vi "Destructor.vi"(8 "error in":errorcluster, 11 "StringMeasureLimit":refnum<class "StringMeasureLimit.lvclass">) -> (0 "error out":errorcluster)   [LabVIEW 2021, in "ProligentXMLGenerator.lvlib" / "StringMeasureLimit.lvclass"]
uses:
  StringMeasureLimit.lvclass
  StringMeasureLimit.lvclass/StringMeasureLimit.ctl
  MeasureLimit/MeasureLimit.lvclass
  C:/Projects/proligent-xml-generator-labview/src/ProligentXMLGenerator/Measure/MeasureLimit/MeasureLimit.lvclass
  C:/Projects/proligent-xml-generator-labview/src/ProligentXMLGenerator/Measure/StringMeasureLimit/StringMeasureLimit.lvclass
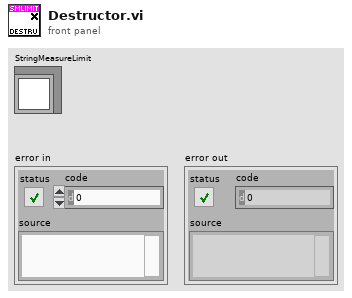
[diagram p1: front panel]
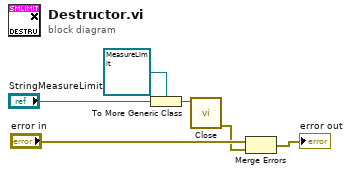
[diagram p0: block diagram]
diagram:
  n1 = To More Generic Class(target class=refnum<class "MeasureLimit.lvclass"> refnum ("ProligentResultProcessor:MeasureLimit"), reference="StringMeasureLimit") -> (generic class reference=w3:refnum<class "MeasureLimit.lvclass">)
  n2 = call "Close.vi"("MeasureLimit"=w3) -> ("error out"=w4:errorcluster)  [unwired: 10 in]
  n3 = Merge Errors("error in", w4) -> (→"error out":errorcluster)
